vi "Servo Close N Channels.vi"(8 "Error In":errorcluster, 10 "Servo Channels":u8[](array[numeric]), 11 "LINX Resource":T1) -> (0 "Error Out":errorcluster, 3 "LINX Resource":T1)   [LabVIEW 2019, in "LMH-LINX.lvlib" / "Servo.lvlib"]
doc: "Read the values of the specified digital input channels."
uses:
  <vilib>/MakerHub/LINX/Public/Sensors/Motion/Servo/Servo.lvlib
  <vilib>/MakerHub/LINX/Private/Type Defs/LINX Ref.ctl
  <vilib>/MakerHub/LINX/Private/Type Defs/Platform.ctl
  <vilib>/MakerHub/LINX/Private/Type Defs/Interface.ctl
  <vilib>/MakerHub/LINX/Private/Device/Type Defs/LINX Device Config.ctl
  <vilib>/MakerHub/LINX/Private/Device/Type Defs/TCP Config.ctl
  <vilib>/MakerHub/LINX/Private/Device/Type Defs/Channels.ctl
  <vilib>/MakerHub/LINX/Private/Type Defs/Peripheral.ctl
  <vilib>/MakerHub/LINX/Private/Type Defs/Error Type.ctl
  <vilib>/MakerHub/LINX/LMH-LINX.lvlib
  <vilib>/MakerHub/LINX/Private/Device/Device.lvlib
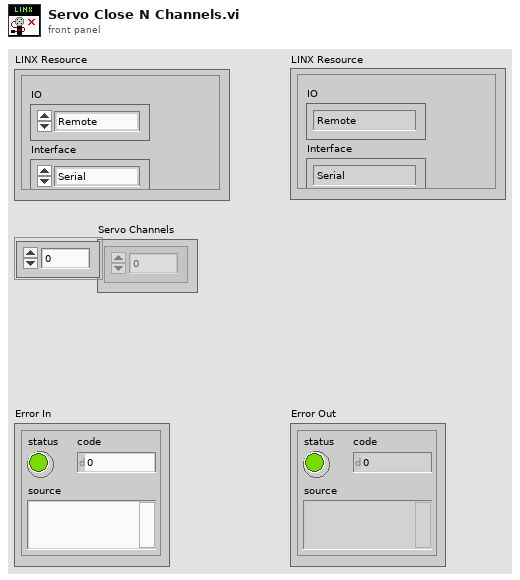
[diagram p1: front panel]
types:
  T1 = typedef "LMH-LINX.lvlib/LINX Ref.ctl" = cluster{"IO":T2, "Interface":T3, "LINX Device Config":T4}
  T2 = typedef "LMH-LINX.lvlib/Platform.ctl" = enum16{"Remote", "Local"}
  T3 = typedef "LMH-LINX.lvlib/Interface.ctl" = enum16{"Serial", "TCP"}
  T4 = typedef "LMH-LINX.lvlib/Device.lvlib/LINX Device Config.ctl" = cluster{"Interface":T3, "COM Port":refnum<visa-resource-name>, "TCP Configuration":T5, "Device Family":u8, "Device ID":u8, "Device Name":string, "TCP Ref":refnum<k5>, "Channels":T6}
  T5 = typedef "LMH-LINX.lvlib/Device.lvlib/TCP Config.ctl" = cluster{"IP Address":string, "Port":u16}
  T6 = typedef "LMH-LINX.lvlib/Channels.ctl" = cluster{"DI":u8[], "DO":u8[], "AI":u8[], "AO":u8[], "PWM":u8[], "QE":u8[], "UART":u8[], "I2C 2":u8[], "SPI":u8[], "CAN":u8[], "Servo":u8[], "AI Ref (V)":dbl, "AI Resolution (Bits)":u8, "AO Ref (V)":dbl, "AO Resolution (Bits)":u8}
  T7 = typedef "LMH-LINX.lvlib/Peripheral.ctl" = enum8{"DI", "DO", "AI", "AO", "PWM", "QE", "UART", "I2C", "SPI", "CAN", "Servo"}
  T8 = typedef "LMH-LINX.lvlib/Error Type.ctl" = enum16{"Unknown", "Timeout", "Corrupt Return Packet", "Unable To Connect", "Command Not Supported", "Channel DNE", "Invalid COM Config", "Firmware Version Mismatch", "myRIO Support", "CMD Specific Error", "Local IO Not Supported"}
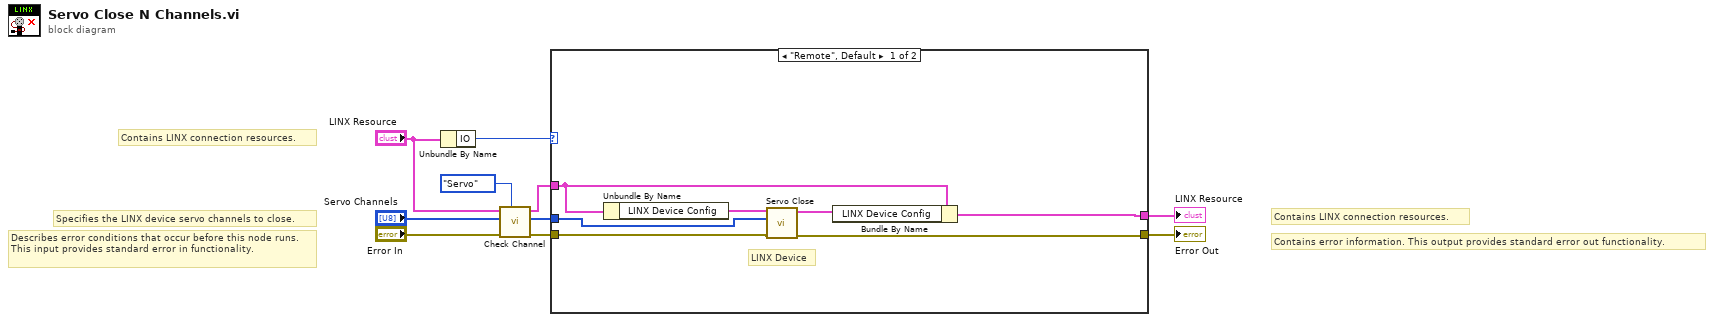
[diagram p0: block diagram]
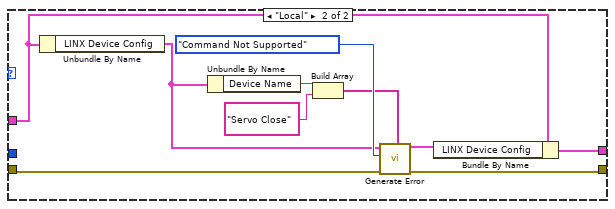
[diagram p2: hidden frame]
diagram:
  # "Specifies the LINX device servo channels to close."
  # "Contains LINX connection resources."
  # "Contains error information. This output provides standard error out functionality."
  # "Contains LINX connection resources."
  # "Describes error conditions that occur before this node runs. This input provides standard error in functionality."
  n1 = Unbundle By Name("LINX Resource") -> ("IO"=w10:T2)
  n2 = call <vilib>:"Check Channel.vi"("Peripheral"=Peripheral."Servo", "Error In"="Error In", "Channels"="Servo Channels", "LINX Resource"="LINX Resource") -> ("Error Out"=w7:errorcluster, "Channels"=w6:u8[], "LINX Resource"=w4:T1)  [unwired: 5 in]
  n3 = case shown="\"Remote\", Default" w10 {
    tunnel: w7 -> [w15 w27]
    tunnel: w4 -> [w17 w20]
    tunnel: [w14 w26] -> w9
    tunnel: [w16 w18] -> w8
    tunnel: w6 -> [w13 _]
    frame "Remote", Default {
      # "LINX Device"
      n4 = Unbundle By Name(w17) -> ("LINX Device Config"=w11:T4)
      n5 = call <vilib>:"Servo Close.vi"("Error In"=w15, "Channels"=w13, "LINX Device Config"=w11) -> ("Error Out"=w14:errorcluster, "LINX Device Config"=w12:T4)  [unwired: 7 in]
      n6 = Bundle By Name(cluster=w17, "LINX Device Config"=w12) -> (w16:T1)
    }
    frame "Local" {
      n7 = Unbundle By Name(w20) -> ("LINX Device Config"=w21:T4)
      n8 = Unbundle By Name(w21) -> ("Device Name"=w25:string)
      n9 = Build Array(w25, "Servo Close") -> (w22:string[])
      n10 = call <vilib>:"Generate Error.vi"("Error In"=w27, "Arguments"=w22, "Error Type"=Error_Type."Command Not Supported", "LINX Device Config"=w21) -> ("Error Out"=w26:errorcluster, "Dup LINX Device Config"=w19:T4)  [unwired: 6 in]
      n11 = Bundle By Name(cluster=w20, "LINX Device Config"=w19) -> (w18:T1)
    }
  }
  "Error Out" <- w9
  "LINX Resource" <- w8
